vi "Turn Left.vi"(6 "Turning angle":sgl=45.0, 10 "Motor B (right)":i8=50, 11 "EV3 in":T1) -> (3 "EV3 out":T1)   [LabVIEW 2015]
uses:
  <vilib>/NXT/Block Support/NXT_InputPort.ctl
  <vilib>/NXT/Dual Mode Library/Sensors/EV3_Gyro_Angle.vi
  <vilib>/NXT/Block Support/NXT_OutputPort.ctl
  <vilib>/NXT/LegoClasses/BrickReference/BrickReference.lvclass
  <vilib>/NXT/Subs/LVHSConnector.ctl
  <vilib>/NXT/NXTIO Xnodes/NXTIOXNode/NXTIO.xnode
  <vilib>/NXT/Dual Mode Library/Waits/Wait_Num.vi
  <vilib>/NXT/NXTIO Xnodes/NXTIONodeSubVIs/NXTMoveMotors.vi
  <vilib>/NXT/NXTIO Xnodes/NXTIONodeSubVIs/NXTStopMotors.vi
  <vilib>/NXT/NXTIO Xnodes/NXTIONodeSubVIs/LEGOResetMotors.vi
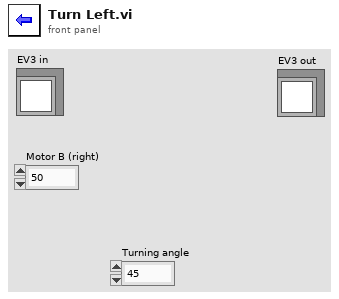
[diagram p1: front panel]
types:
  T1 = typedef "LVHSConnector.ctl" = refnum<class "BrickReference.lvclass">
  T2 = typedef "NXT_OutputPort.ctl" = u8
  T3 = typedef "NXT_InputPort.ctl" = u32
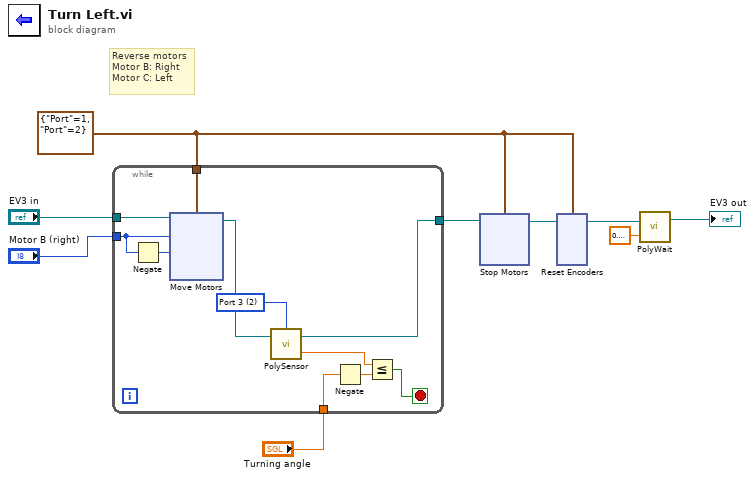
[diagram p0: block diagram]
diagram:
  w4 = cluster{"Port":T2, "Port":T2} {"Port"=1, "Port"=2} ("Motor")
  # "Reverse motors\nMotor B: Right\nMotor C: Left"
  n1 = while {
    tunnel: [w16] -> w6
    tunnel: "EV3 in" -> [w15]
    tunnel: w4 -> [w14]
    tunnel: "Turning angle" -> [w13]
    tunnel: "Motor B (right)" -> [w10]
    stop <- w19 stop-if-true
    w18 = T3 2 items=["Port 1", "Port 2", "Port 3", "Port 4"] ("Port (Port 1)")
    n2 = Negate(x=w10) -> (-x=w12:i8)
    n3 = xnode "Move Motors"("Power/Speed 2"=w12, "Power/Speed 1"=w10, "Motors"=w14, "NXT/EV3"=w15) -> ("NXT/EV3"=w17:T1)
    n4 = call-poly <vilib>:"PolySensor.vi"("NXT/EV3"=w17, "Port (Port 1)"=w18) -> ("Degrees"=w20:sgl, "NXT/EV3"=w16:T1)  [unwired: 1 in]
    n5 = Negate(x=w13) -> (-x=w11:sgl)
    n6 = Less Or Equal?(x=w20, y=w11) -> (x <= y?=w19:bool)
  }
  n7 = xnode "Stop Motors"("Motors"=w4, "NXT/EV3"=w6) -> ("NXT/EV3"=w5:T1)
  n8 = xnode "Reset Encoders"("Motors"=w4, "NXT/EV3"=w5) -> ("NXT/EV3"=w2:T1)
  n9 = call-poly <vilib>:"PolyWait.vi"("Time (1 sec)"=sgl 0.2, "NXT/EV3"=w2) -> ("NXT/EV3"=→"EV3 out":T1)  [unwired: 2 in]
